vi "Test Launch Dim UI.vi"   [LabVIEW 2020, in "Better Search.lvlib" / "BetterSearch.lvclass"]
uses:
  BetterSearch.lvclass
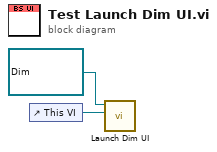
[diagram p0: block diagram]
diagram:
  n1 = control-ref of="This VI"() -> (w2:refnum<vi>)
  n2 = call "Launch Dim UI.vi"("From VI"=w2, "Dim UI"=refnum<user-event> refnum) -> ()  [unwired: 9 in, 1 out]
